vi "Servo MSMT WCDMA Set DC Params.vi"(8 "error in (no error)":errorcluster, 10 "Step In":refnum<k7>, 11 "Servo MSMT in":refnum<class "Servo MSMT.lvclass">) -> (0 "error out":errorcluster, 2 "Step Out":refnum<k7>, 3 "Servo MSMT out":refnum<class "Servo MSMT.lvclass">)   [LabVIEW 2018, in "Servo MSMT.lvlib" / "Servo MSMT.lvclass"]
uses:
  Servo MSMT.lvclass
  Servo MSMT.lvclass/Servo MSMT.ctl
  Protected Methods/Read DC Pins.vi
  C:/Sequence Automation/Plugins/Measurement Interface.lvlibp/Measurement Interface.lvclass
  Plugins/Measurement Interface.lvlibp/Measurement Interface.lvclass
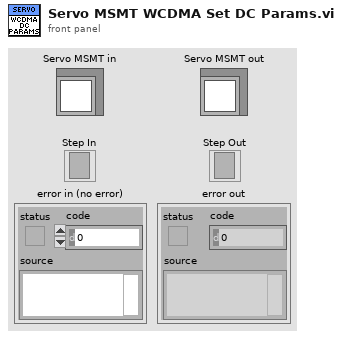
[diagram p1: front panel]
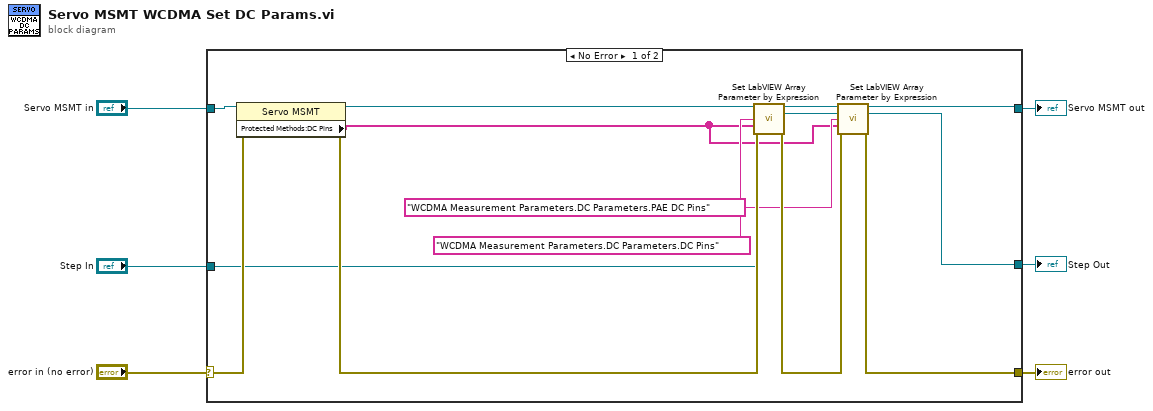
[diagram p0: block diagram]
diagram:
  n1 = case shown="No Error" "error in (no error)" {
    selector: "error in (no error)" -> [w20 w23]
    tunnel: [w15 w23] -> w5
    tunnel: [w8 w22] -> w3
    tunnel: "Servo MSMT in" -> [w19 w22]
    tunnel: "Step In" -> [w13 w21]
    tunnel: [w12 w21] -> w1
    frame No Error {
      n2 = property class="Servo MSMT"(reference=w19, error in=w20) -> (reference out=w10:refnum<class "Servo MSMT.lvclass">, error out=w18:errorcluster, "Protected Methods:DC Pins"=w7:string[])
      n3 = call "Set LabVIEW Array Parameter by Expression.vi"("Measurement Interface in"=w10, "Step In"=w13, "LabVIEW Parameter to Set"="WCDMA Measurement Parameters.DC Parameters.DC Pins", "Array of Expresssions"=w7, "error in (no error)"=w18) -> ("Measurement Interface out"=w9:refnum<class "Servo MSMT.lvclass">, "Step Out"=w14:refnum<k7>, "error out"=w16:errorcluster)  [unwired: 8 in]
      n4 = call "Set LabVIEW Array Parameter by Expression.vi"("Measurement Interface in"=w9, "Step In"=w14, "LabVIEW Parameter to Set"="WCDMA Measurement Parameters.DC Parameters.PAE DC Pins", "Array of Expresssions"=w7, "error in (no error)"=w16) -> ("Measurement Interface out"=w8:refnum<class "Servo MSMT.lvclass">, "Step Out"=w12:refnum<k7>, "error out"=w15:errorcluster)  [unwired: 8 in]
    }
    frame Error {
    }
  }
  "error out" <- w5
  "Servo MSMT out" <- w3
  "Step Out" <- w1
